vi "test Loopback BC to RT with Acyclic Frame.vi"(8 "error in":errorcluster, 11 "TestCase in":refnum<class "Loopback.lvclass">) -> (0 "error out":errorcluster, 3 "TestCase out":refnum<class "Loopback.lvclass">)   [LabVIEW 2020, in "Loopback.lvclass"]
uses:
  Loopback.lvclass
  C:/Git/niveristand-custom-device-testing-tools/VeriStandTestCase/VeriStandTestCase.lvclass
  <vilib>/NI VeriStand/Execution/Workspace/NI VeriStand - Set Single Channel Value.vi
  <vilib>/addons/_JKI Toolkits/VI Tester/TestCase.llb/TestCase.lvclass
  <vilib>/NI VeriStand/Execution/Workspace/NI_VS Workspace ExecutionAPI.lvlib
  niveristand-custom-device-testing-tools/VeriStandTestUtilities/VeriStandTestUtilities.lvlib
  C:/Program Files (x86)/National Instruments/LabVIEW 2020/vi.lib/addons/_JKI Toolkits/VI Tester/TestCase.llb/TestCase.lvclass
  C:/Git/niveristand-ballard-milStd1553-custom-device/Source/Custom Device Support/Tests/System/Loopback/Loopback.lvclass
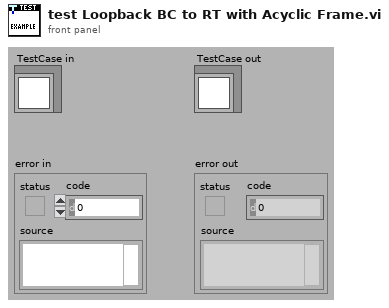
[diagram p1: front panel]
types:
  T1 = typedef "NI_VS Workspace ExecutionAPI.lvlib/WorkspaceAPI.ctl" = refnum<k24>
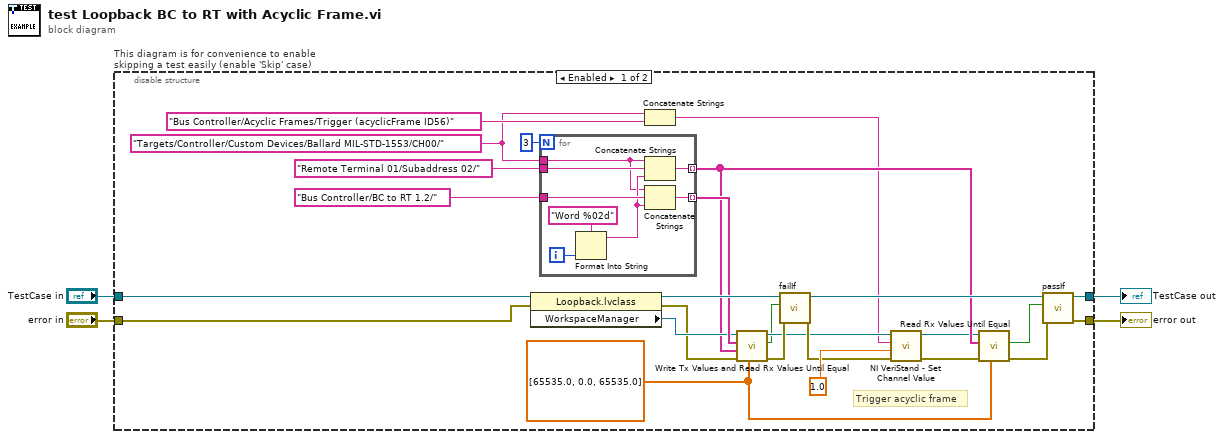
[diagram p0: block diagram]
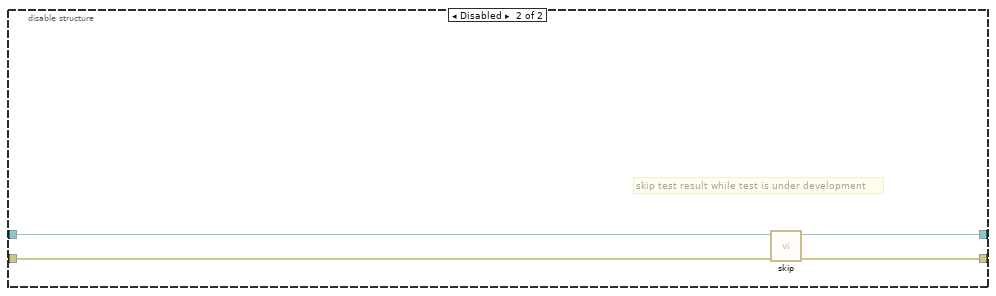
[diagram p2: hidden frame]
diagram:
  n1 = disable-structure "This diagram is for convenience to enable skipping a test easily (enable 'Skip' case)" shown="Enabled" {
    disable-tunnel: "TestCase in" -> [w30 w42]
    disable-tunnel: [w23 w40] -> w1
    disable-tunnel: [w21 w41] -> w3
    disable-tunnel: "error in" -> [w29 w39]
    frame Enabled {
      w6 = "Targets/Controller/Custom Devices/Ballard MIL-STD-1553/CH00/" ("Channel")
      w8 = dbl[] [65535.0, 0.0, 65535.0]
      # "Trigger acyclic frame"
      n2 = property class="Loopback.lvclass"(reference=w30, error in=w29) -> (reference out=w20:refnum<class "Loopback.lvclass">, error out=w17:errorcluster, "WorkspaceManager"=w18:T1)
      n3 = for {
        N: 3 -> [_]
        tunnel: "Bus Controller/BC to RT 1.2/" ("Channel") -> [w37]
        tunnel: [w38] -> w19 mode=indexing
        tunnel: "Remote Terminal 01/Subaddress 02/" ("Channel") -> [w36]
        tunnel: [w35] -> w15 mode=indexing
        tunnel: w6 -> [w31]
        i -> [w34]
        n4 = Format Into String(format string="Word %02d", w34) -> (resulting string=w33:string)  [unwired: 2 in, 1 out]
        n5 = Concatenate Strings(w31, w36, w33) -> (w35:string)
        n6 = Concatenate Strings(w31, w37, w33) -> (w38:string)
      }
      n7 = Concatenate Strings(w6, "Bus Controller/Acyclic Frames/Trigger (acyclicFrame ID56)") -> (w5:string)
      n8 = call "Write Tx Values and Read Rx Values Until Equal.vi"("Tx values"=w8, "error in"=w17, "Rx aliases"=w15, "Tx aliases"=w19, "workspace manager in"=w18) -> ("error out"=w16:errorcluster, "values equal"=w9:bool, "workspace manager out"=w13:T1)  [unwired: 4 in]
      n9 = call-dynamic "failIf.vi"("error in (no error)"=w16, "fail"=w9, "TestCase in"=w20) -> ("error out"=w24:errorcluster, "TestCase out"=w22:refnum<class "Loopback.lvclass">)  [unwired: 7 in]
      n10 = call-poly <vilib>:"NI VeriStand - Set Channel Value.vi"("error in (no error)"=w24, "Value"=1.0, "Channel"=w5, "WorkspaceManager in"=w13) -> ("error out"=w10:errorcluster, "WorkspaceManager out"=w11:T1)  [unwired: 6 in]
      n11 = call "Read Rx Values Until Equal.vi"("expected values"=w8, "error in"=w10, "Rx aliases"=w15, "workspace manager in"=w11) -> ("error out"=w12:errorcluster, "values equal expected"=w14:bool)  [unwired: 5 in, 1 out]
      n12 = call-dynamic "passIf.vi"("error in (no error)"=w12, "pass"=w14, "TestCase in"=w22) -> ("error out"=w21:errorcluster, "TestCase out"=w23:refnum<class "Loopback.lvclass">)  [unwired: 7 in]
    }
    frame Disabled {
      # "skip test result while test is under development"
      n13 = call <vilib>:"skip.vi"("error in (no error)"=w39, "TestCase in"=w42) -> ("error out"=w41:errorcluster, "TestCase out"=w40:refnum<class "Loopback.lvclass">)  [unwired: 8 in]
    }
  }
  "error out" <- w3
  "TestCase out" <- w1
